vi "MB Modbus Demo Box Example (Legacy).vi"() -> ()   [LabVIEW 2011]
uses:
  MB Modbus Command.ctl
panel:
  in  "Ouputs":u16[](array[slide]) max=60 scale=0.0..60.0
  in  "Digital Outputs":T1
  out "Analog Inputs":T2 {"AI 5" scale=0.0..100.0; "AI 4" scale=0.0..100.0; "AI 3" scale=0.0..100.0; "AI 2" scale=0.0..100.0; "AI 1" scale=0.0..100.0}
  out "Digital Inputs":T3
  in  "COM Port":refnum<visa-resource-name>
  in  "Power":bool
  out "Power LED":bool
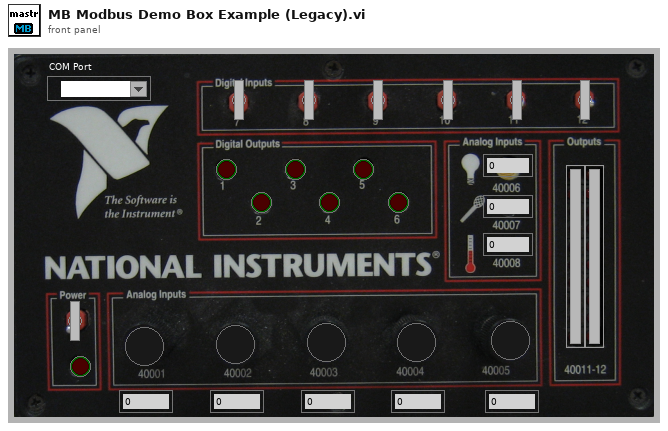
[diagram p1: front panel]
types:
  T1 = cluster{"DO 1":bool, "DO 2":bool, "DO 3":bool, "DO 4":bool, "DO 5":bool, "DO 6":bool}
  T2 = cluster{"AI 1":u16, "AI 2":u16, "AI 3":u16, "AI 4":u16, "AI 5":u16, "40006":u16, "40007":u16, "40008":u16}
  T3 = cluster{"DI1":bool, "DI1 2":bool, "DI1 3":bool, "DI1 4":bool, "DI1 5":bool, "DI1 6":bool}
  T4 = cluster{"Mode":enum16{"RTU", "ASCII"}, "Slave Address":u8}
  T5 = typedef "MB Modbus Command.ctl" = cluster{"Function Code":u8, "Starting Address":u16, "Quantity":u16, "Data":u16[], "Discrete":bool[]}
  T6 = cluster{"Discrete[0]":bool, "Discrete[1]":bool, "Discrete[2]":bool, "Discrete[3]":bool, "Discrete[4]":bool, "Discrete[5]":bool}
  T7 = cluster{"Registers[0]":u16, "Registers[1]":u16, "Registers[2]":u16, "Registers[3]":u16, "Registers[4]":u16, "Registers[5]":u16, "Registers[6]":u16, "Registers[7]":u16}
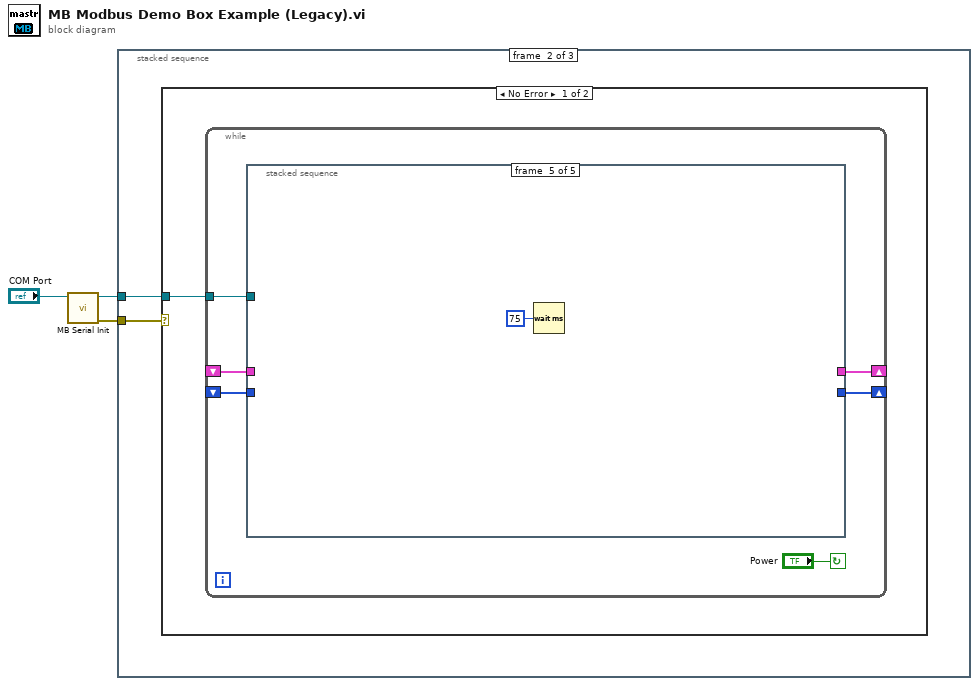
[diagram p0: block diagram]
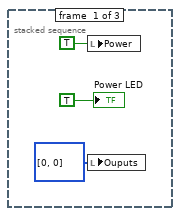
[diagram p2: hidden frame]
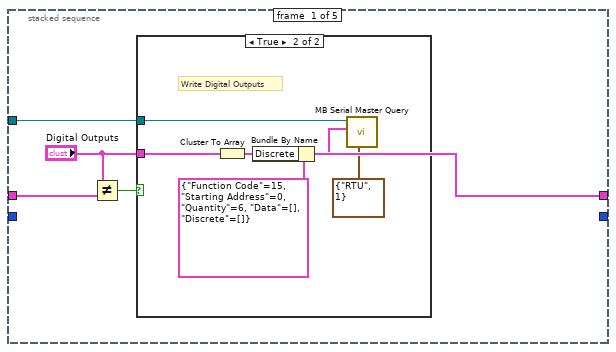
[diagram p3: hidden frame]
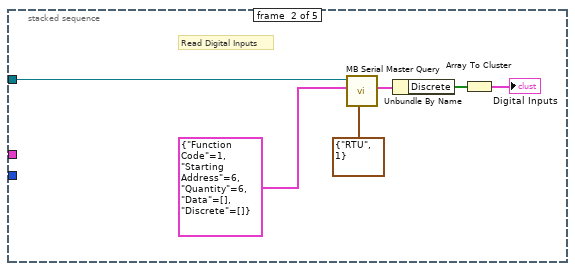
[diagram p5: hidden frame]
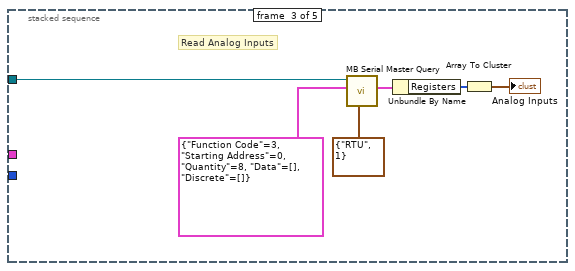
[diagram p6: hidden frame]
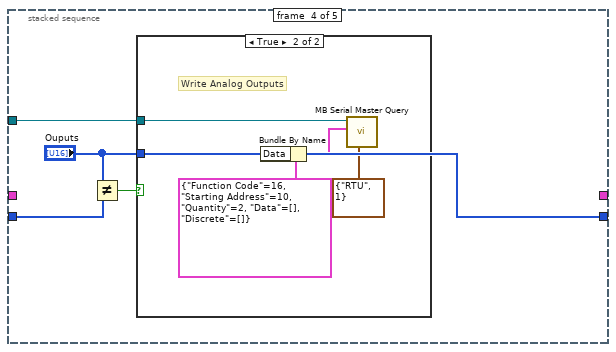
[diagram p7: hidden frame]
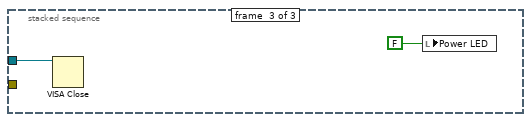
[diagram p10: hidden frame]
diagram:
  n1 = call "MB Serial Init.vi"("VISA resource name"="COM Port") -> ("error out"=w1:errorcluster, "VISA resource name out"=w2:refnum<visa-resource-name>)  [unwired: 6 in, 3 out]
  n2 = stacked-sequence {
    tunnel: w2 -> [_ w8 w48]
    tunnel: w1 -> [_ w7 _]
    frame #0 {
      n3 = local write "Power"(TRUE ("Power")) -> ()
      n4 = local write "Ouputs"(u16[] [0, 0] ("Ouputs")) -> ()
      "Power LED" <- TRUE ("Power LED")
    }
    frame #1 {
      n5 = case shown="No Error" w7 {
        tunnel: w8 -> [w9 _]
        frame No Error {
          n6 = while {
            shift-right: [w12] -> _
            shift-left: _ -> [w15]
            tunnel: w9 -> [w14]
            shift-right: [w11] -> _
            shift-left: _ -> [w13]
            stop <- "Power" continue-if-true
            n7 = stacked-sequence {
              tunnel: w15 -> [w18 _ _ _ _]
              tunnel: w14 -> [w17 w26 w32 w40 _]
              tunnel: w13 -> [_ _ _ w39 _]
              tunnel: ["Digital Outputs" _ _ _ _] -> w12
              tunnel: [_ _ _ "Ouputs" _] -> w11
              frame #0 {
                n8 = Not Equal?(x="Digital Outputs", y=w18) -> (x != y?=w19:bool)
                n9 = case shown="True" w19 {
                  tunnel: "Digital Outputs" -> [_ w21]
                  tunnel: w17 -> [_ w20]
                  frame False {
                  }
                  frame True {
                    # "Write Digital Outputs"
                    n10 = Cluster To Array(cluster=w21) -> (array=w24:bool[])
                    n11 = Bundle By Name(cluster=T5 {"Function Code"=15, "Starting Address"=0, "Quantity"=6, "Data"=[], "Discrete"=[]} ("MODBUS Command"), "Discrete"=w24) -> (w22:T5)
                    n12 = call "MB Serial Master Query.vi"("Serial Parameters"=T4 {"Mode"=enum."RTU", "Slave Address"=1}, "Modbus Command"=w22, "VISA resource name"=w20) -> ()  [unwired: 4 in, 5 out]
                  }
                }
              }
              frame #1 {
                # "Read Digital Inputs"
                n13 = call "MB Serial Master Query.vi"("Serial Parameters"=T4 {"Mode"=enum."RTU", "Slave Address"=1}, "Modbus Command"=T5 {"Function Code"=1, "Starting Address"=6, "Quantity"=6, "Data"=[], "Discrete"=[]} ("MODBUS Command"), "VISA resource name"=w26) -> ("Registers"=w31:cluster{"Registers":u16[], "Discrete":bool[]})  [unwired: 4 in, 4 out]
                n14 = Unbundle By Name(w31) -> ("Discrete"=w28:bool[])
                n15 = Array To Cluster(array=w28) -> (cluster=→"Digital Inputs":T6)
              }
              frame #2 {
                # "Read Analog Inputs"
                n16 = call "MB Serial Master Query.vi"("Serial Parameters"=T4 {"Mode"=enum."RTU", "Slave Address"=1}, "Modbus Command"=T5 {"Function Code"=3, "Starting Address"=0, "Quantity"=8, "Data"=[], "Discrete"=[]} ("MODBUS Command"), "VISA resource name"=w32) -> ("Registers"=w37:cluster{"Registers":u16[], "Discrete":bool[]})  [unwired: 4 in, 4 out]
                n17 = Unbundle By Name(w37) -> ("Registers"=w34:u16[])
                n18 = Array To Cluster(array=w34) -> (cluster=→"Analog Inputs":T7)
              }
              frame #3 {
                n19 = Not Equal?(x="Ouputs", y=w39) -> (x != y?=w41:bool)
                n20 = case shown="True" w41 {
                  tunnel: "Ouputs" -> [_ w42]
                  tunnel: w40 -> [_ w43]
                  frame False {
                  }
                  frame True {
                    # "Write Analog Outputs"
                    n21 = Bundle By Name(cluster=T5 {"Function Code"=16, "Starting Address"=10, "Quantity"=2, "Data"=[], "Discrete"=[]} ("MODBUS Command"), "Data"=w42) -> (w44:T5)
                    n22 = call "MB Serial Master Query.vi"("Serial Parameters"=T4 {"Mode"=enum."RTU", "Slave Address"=1}, "Modbus Command"=w44, "VISA resource name"=w43) -> ()  [unwired: 4 in, 5 out]
                  }
                }
              }
              frame #4 {
                n23 = Wait (ms)(milliseconds to wait=u32 75) -> ()  [unwired: 1 out]
              }
            }
          }
        }
        frame Error {
        }
      }
    }
    frame #2 {
      n24 = VISA Close(VISA resource name=w48) -> ()  [unwired: 1 in, 1 out]
      n25 = local write "Power LED"(FALSE ("Power LED")) -> ()
    }
  }
